vi "Get Harmonic.vi"(8 "error in (no error)":errorcluster, 11 "VISA resource name":refnum<visa-resource-name>) -> (0 "error out":errorcluster, 1 "Fundamental":u16, 2 "Harmonic Value":i32, 3 "VISA resource name out":refnum<visa-resource-name>)   [LabVIEW 2011, in "Fluke 5XXX Series Multicalibrators.lvlib"]
doc: "Returns the present instrument harmonic characteristic and location of the fundamental output Primary (the NORMAL terminals) or Secondary (the AUX terminals).\n\nNote:\n\nThis VI is available only for instrument models 5500A and 5520A."
uses:
  Fluke 5XXX Series Multicalibrators.lvlib
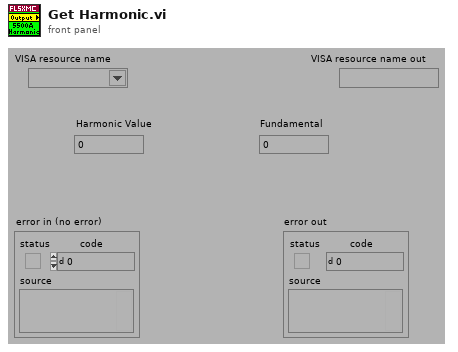
[diagram p1: front panel]
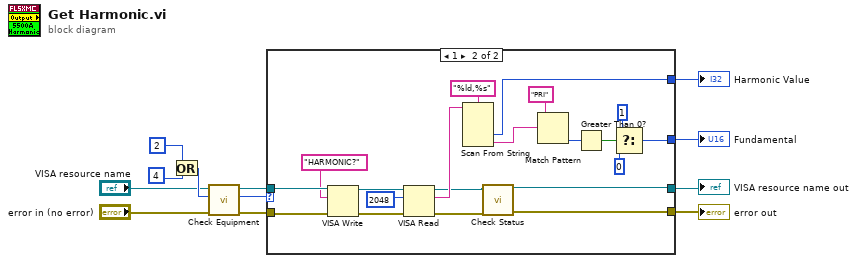
[diagram p0: block diagram]
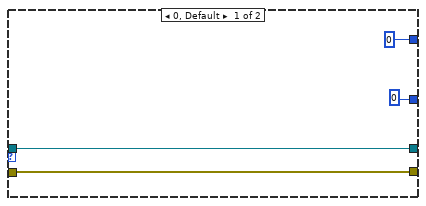
[diagram p2: hidden frame]
diagram:
  n1 = Or(x=2 ("Numeric"), y=4 ("Numeric")) -> (x .or. y?=w9:i32)
  n2 = call "Check Equipment.vi"("error in (no error)"="error in (no error)", "Bit Mask"=w9, "VISA resource name"="VISA resource name") -> ("error out"=w12:errorcluster, "Present?"=w11:u32, "VISA resource name out"=w10:refnum<visa-resource-name>)  [unwired: 6 in]
  n3 = case shown="1" w11 {
    tunnel: [w15 w35] -> w5
    tunnel: w12 -> [w16 w34]
    tunnel: w10 -> [w15 w33]
    tunnel: [w16 w36] -> w6
    tunnel: [0 w24] -> w1
    tunnel: [u16 0 ("f") w18] -> w2
    frame 0, Default {
    }
    frame 1 {
      n4 = VISA Write(VISA resource name=w33, write buffer="HARMONIC?", error in (no error)=w34) -> (VISA resource name out=w30:refnum<visa-resource-name>, error out=w29:errorcluster)  [unwired: 1 out]
      n5 = VISA Read(VISA resource name=w30, byte count=u32 2048 ("byte count (0)"), error in (no error)=w29) -> (VISA resource name out=w25:refnum<visa-resource-name>, read buffer=w26:string, error out=w27:errorcluster)  [unwired: 1 out]
      n6 = Scan From String(format string="%ld,%s", input string=w26) -> (output 1=w24:i32, output 2=w23:string)  [unwired: 4 in, 3 out]
      n7 = call "Check Status.vi"("VISA resource name"=w25, "error in (no error)"=w27) -> ("VISA resource name out"=w35:refnum<visa-resource-name>, "error out"=w36:errorcluster)  [unwired: 12 in]
      n8 = Match Pattern(string=w23, regular expression="PRI") -> (offset past match=w21:i32)  [unwired: 1 in, 3 out]
      n9 = Greater Than 0?(x=w21) -> (x > 0?=w17:bool)
      n10 = Select(t=u16 1 ("f"), s=w17, f=u16 0) -> (s? t:f=w18:u16)
    }
  }
  "Harmonic Value" <- w1
  "Fundamental" <- w2
  "VISA resource name out" <- w5
  "error out" <- w6
